vi "Submodule EOL UI.vi"() -> ()   [LabVIEW 2025, in "Submodule EOL.lvlib" / "Submodule EOL.lvclass"]
doc: "Copyright 2017 National Instruments Corporation\n\nLicensed under the Apache License, Version 2.0 (the \"License\"); you may not use this file except in compliance with the License. You may obtain a copy of the License at http://www.apache.org/licenses/LICENSE-2.0\nUnless required by applicable law or agreed to in writing, software distributed under the License is distributed on an \"AS IS\" BASIS, WITHOUT WARRANTIES OR CONDITIONS OF ANY KIND, either express or implied. See the License for the specific language governing permissions and limitations under the License."
uses:
  Submodule EOL.lvclass
  Users/Public/Documents/Sandia National Labs/TSS Plugin/CEF.lvlibp/Node/mainQref.ctl
  Users/Public/Documents/Sandia National Labs/TSS Plugin/CEF.lvlibp/Node/UserEventRef.ctl
  Submodule EOL configuration/Submodule EOL.ctl
  Users/Public/Documents/Sandia National Labs/TSS Plugin/CEF.lvlibp/Node/NodeRef.ctl
  Users/Public/Documents/Sandia National Labs/TSS Plugin/CEF.lvlibp/Node/CEF_Node.lvclass
  C:/Users/Public/Documents/Sandia National Labs/TSS Plugin/CEF.lvlibp/Node/CEF_Node.lvclass
  Users/Public/Documents/Sandia National Labs/TSS Plugin/Abstract Engine.lvlibp/Abstract Instrument/Abstract Instrument.lvclass
  Submodule EOL.lvclass/Submodule EOL.ctl
  Submodule EOL configuration/Submodule EOL configuration.lvclass/Submodule EOL configuration.ctl
  <vilib>/Utility/miscctls.llb/LVPositionTypeDef.ctl
  Users/Public/Documents/Sandia National Labs/TSS Plugin/Engines/DMM.lvlibp/DMM Instrument/DMM Instrument.lvclass
  C:/Users/Public/Documents/Sandia National Labs/TSS Plugin/Abstract Engine.lvlibp/Abstract Instrument/Abstract Instrument.lvclass
  Users/Public/Documents/Sandia National Labs/TSS Plugin/Engines/ACIR.lvlibp/ACIR Instrument/ACIR Instrument.lvclass
  Users/Public/Documents/Sandia National Labs/TSS Plugin/Engines/HiPOT.lvlibp/HiPOT Instrument/HiPOT Instrument.lvclass
  Users/Public/Documents/Sandia National Labs/TSS Plugin/Engines/Digital IO.lvlibp/Digital IO Instrument/Digital IO Instrument.lvclass
  Submodule EOL configuration/Read Submodule EOL.vi
  Submodule EOL configuration/Write Submodule EOL.vi
  Submodule EOL configuration/Submodule EOL configuration.lvclass
panel:
  in  "node ref":T1
  in  "Sequence":cluster{"Sequence":string}
  out "Data":T2 {"HiPOT Channels"."Measurement" format="%#_4p"; "ACIR Channels"."Measurement" format="%#_4p"; "DMM Channels"."Measurement" format="%#_4p"}
  in  "Segmented":enum32{"Setting", "Data", "Sequence"}(radio)
  in  "Submodule EOL":T3={"PLC Folder Names"=[], "Timeout Connect OPC"=0.0, "Connect OPC Trial"=0, "PLC URL"="", "Digitial IO"="", "HiPOT"="", "ACIR with Switch"="", "DMM with Switch"="", "Ignition Folder Names"=[], "Ignition URL"="", "Test Name"="Battery Submodule End of Line"} {"Timeout Connect OPC" format="%#_f"}
  in  "user event":T4
  in  "main queue":T5
  # "ch"
  # "ch"
  # "ch"
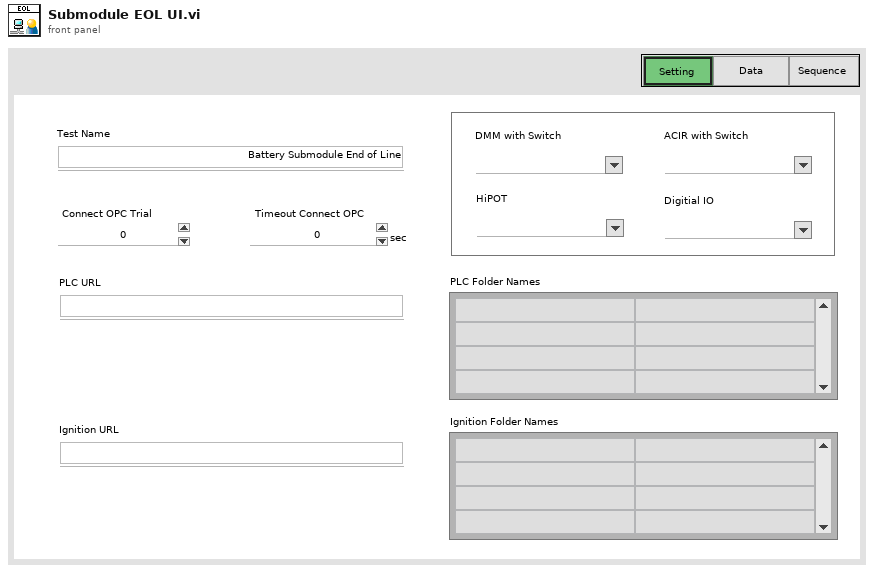
[diagram p1: front panel]
types:
  T1 = typedef "CEF.lvlibp/CEF_Node.lvclass/NodeRef.ctl" = refnum<data-value>
  T2 = cluster{"DMM Channels":cluster{"Channel Alias":string, "Index":i32, "Measurement":dbl}[], "ACIR Channels":cluster{"Channel Alias":string, "Index":i32, "Measurement":dbl}[], "HiPOT Channels":cluster{"Channel Alias":string, "Index":i32, "Measurement":dbl}[], "Digital IO":bool[]}
  T3 = typedef "Submodule EOL.lvlib/Submodule EOL configuration.lvclass/Submodule EOL.ctl" = cluster{"PLC Folder Names":string[][], "Timeout Connect OPC":dbl, "Connect OPC Trial":u32, "PLC URL":string, "Digitial IO":string, "HiPOT":string, "ACIR with Switch":string, "DMM with Switch":string, "Ignition Folder Names":string[][], "Ignition URL":string, "Test Name":string}
  T4 = typedef "CEF.lvlibp/CEF_Node.lvclass/UserEventRef.ctl" = refnum<user-event>
  T5 = typedef "CEF.lvlibp/CEF_Node.lvclass/mainQref.ctl" = refnum<queue>
  T6 = cluster{"Channel Alias":string, "Index":i32, "Measurement":dbl}
  T7 = cluster{"Channel":string, "Index":i32, "Measure":dbl}
  T8 = typedef "LVPositionTypeDef.ctl" = cluster{"Left":i32, "Top":i32}
  T9 = typedef "Abstract Engine.lvlibp/Abstract Instrument.lvclass/Channel.ctl" = cluster{"Alias":string, "DataType":enum16{"Anaolg Input", "Waveform"}, "Unit":enum16{"---", "V", "A", "Ohm", "Hz", "uF", "degC", "deg"}, "Upper limit":dbl, "Lower limit":dbl, "Measurement":variant}
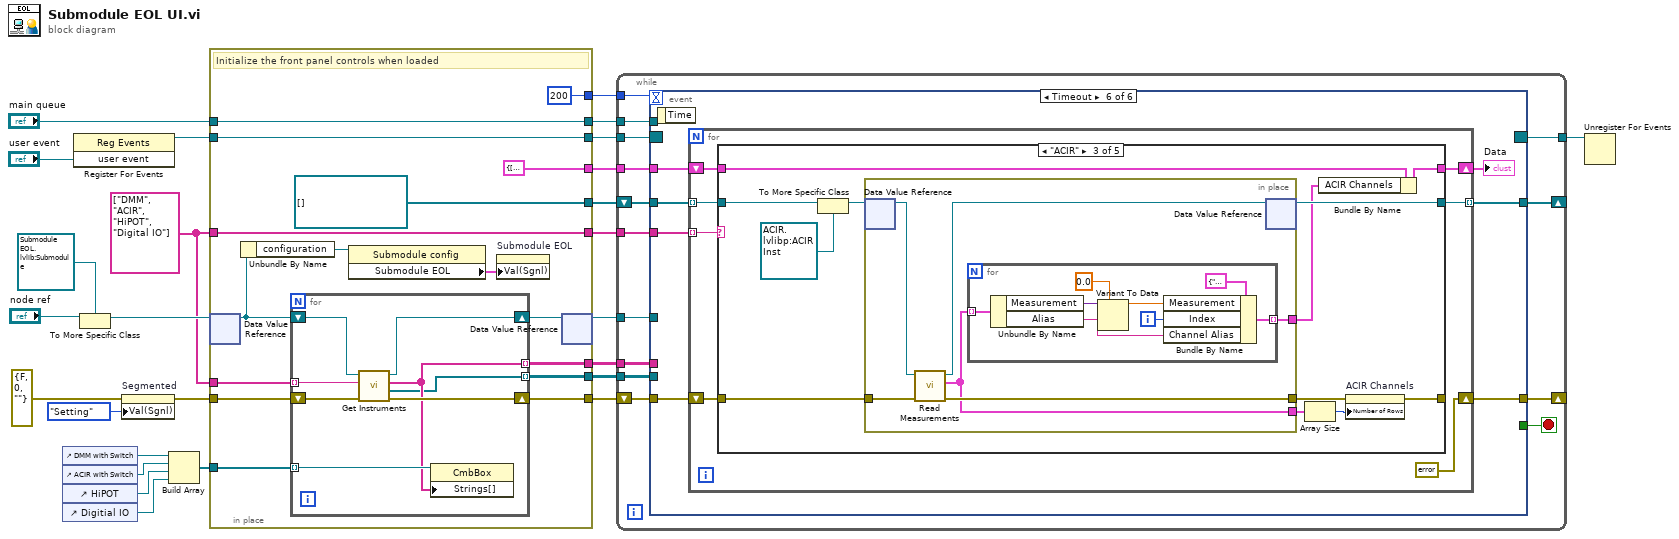
[diagram p0: block diagram]
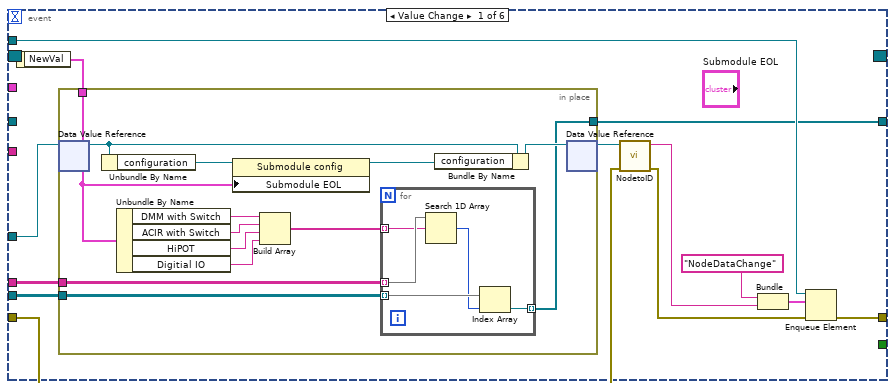
[diagram p2: hidden frame]
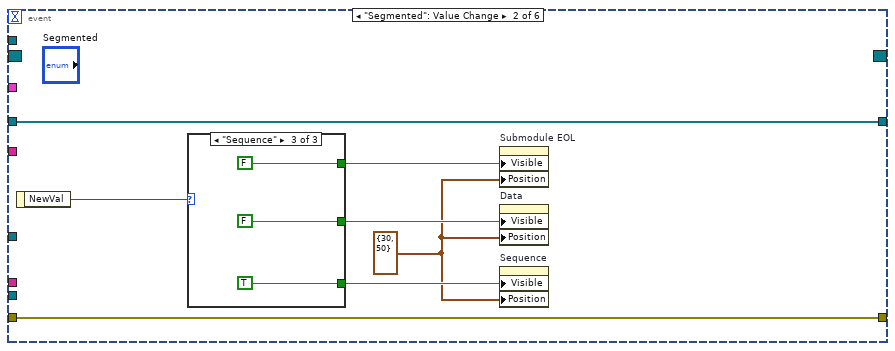
[diagram p3: hidden frame]
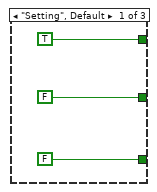
[diagram p4: hidden frame]
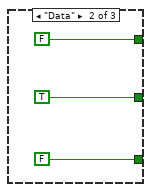
[diagram p5: hidden frame]
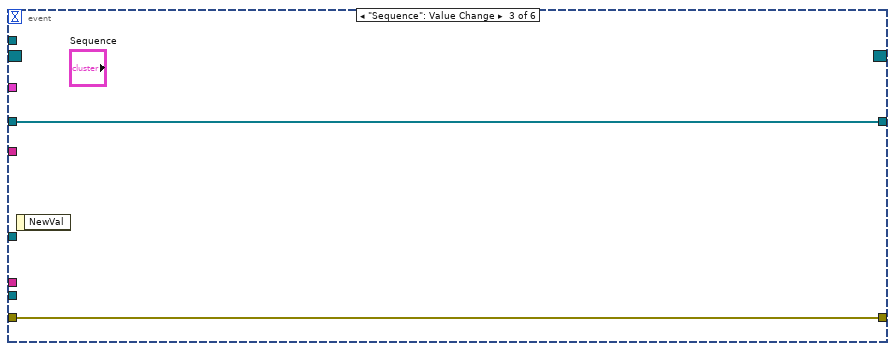
[diagram p6: hidden frame]
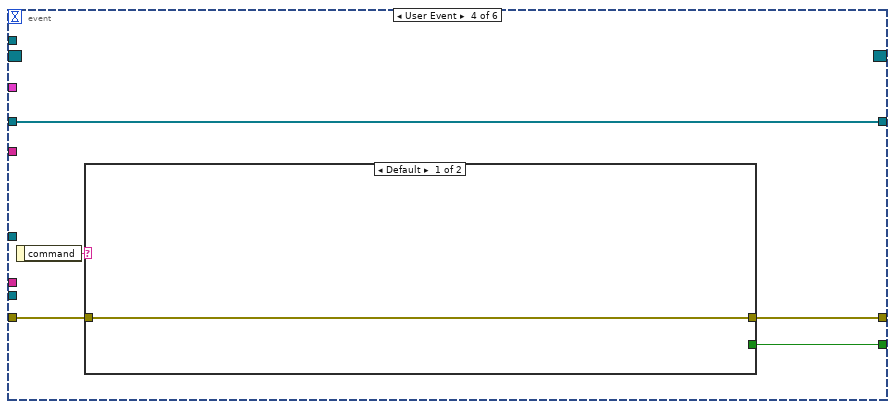
[diagram p7: hidden frame]
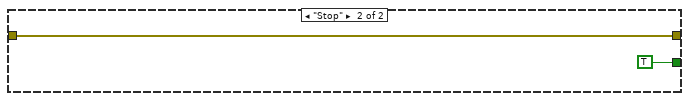
[diagram p8: hidden frame]
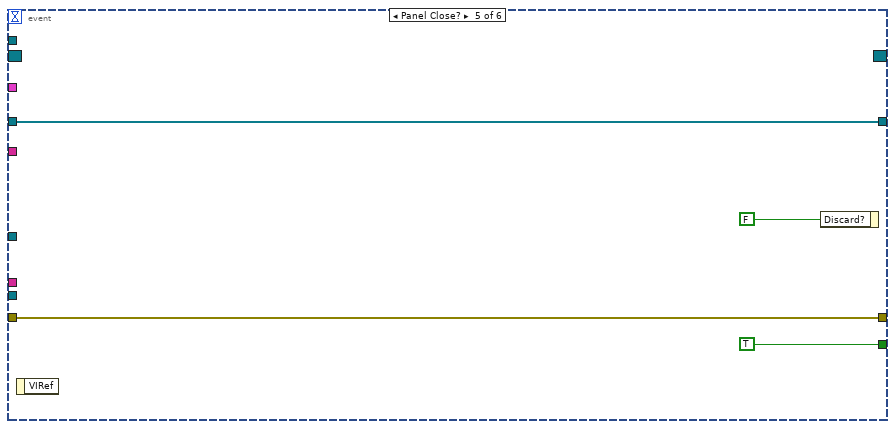
[diagram p9: hidden frame]
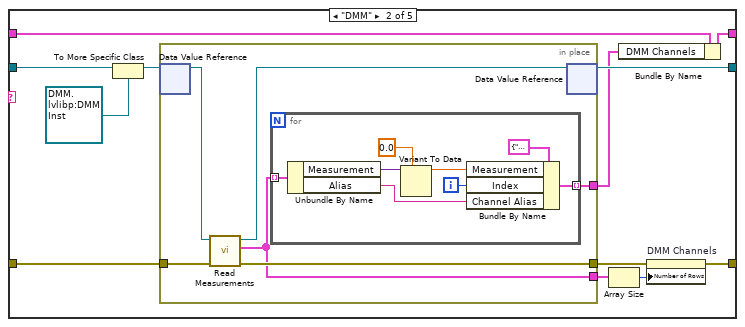
[diagram p11: hidden frame]
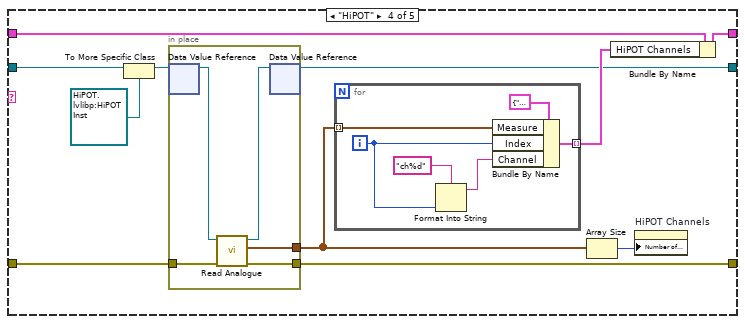
[diagram p12: hidden frame]
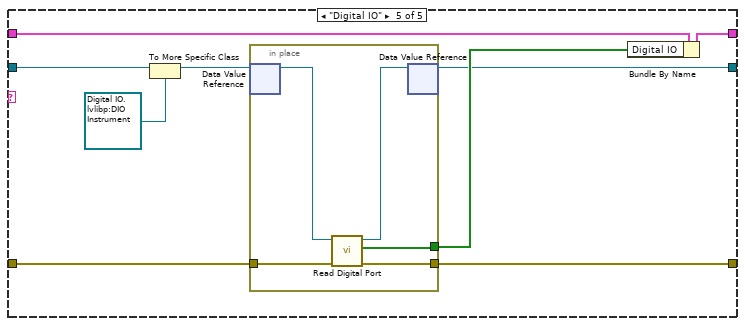
[diagram p13: hidden frame]
diagram:
  w13 = string[] ["DMM", "ACIR", "HiPOT", "Digital IO"]
  n1 = control-ref of="DMM with Switch"() -> (w21:refnum<vi>)
  n2 = control-ref of="ACIR with Switch"() -> (w22:refnum<vi>)
  n3 = control-ref of="HiPOT"() -> (w23:refnum<vi>)
  n4 = control-ref of="Digitial IO"() -> (w24:refnum<vi>)
  n5 = register-events("user event") -> (reference out=w4:refnum<event-registration>)  [unwired: 2 in, 1 out]
  n6 = To More Specific Class(target class=refnum<data-value> refnum ("data value reference"), reference="node ref") -> (specific class reference=w15:refnum<data-value>)  [unwired: 1 in, 1 out]
  n7 = property on="Segmented" class="RadioBtnsControl (strict)"(error in=errorcluster {"status"=FALSE, "code"=0, "source"=""} ("error out"), "Val(Sgnl)"=enum32{"Setting", "Data", "Sequence"}."Setting" ("Segmented Control")) -> (error out=w8:errorcluster)  [unwired: 1 in, 1 out]
  n8 = Build Array(w21, w22, w23, w24) -> (w20:refnum<vi>[])
  n9 = in-place {
    in-place-border: w13 -> [w39]
    in-place-border: w20 -> [w41]
    in-place-border: [w32] -> w6
    in-place-border: "main queue" -> [w40]
    in-place-border: [w40] -> w18
    in-place-border: [w38] -> w17
    in-place-border: [w37] -> w16
    in-place-border: w8 -> [w36]
    in-place-border: [refnum<data-value>[] []] -> w14
    in-place-border: w13 -> [w29]
    in-place-border: [w29] -> w7
    in-place-border: [200] -> w12
    in-place-border: [T2 {"DMM Channels"=[], "ACIR Channels"=[], "HiPOT Channels"=[], "Digital IO"=[]} ("Data")] -> w11
    in-place-border: w4 -> [w30]
    in-place-border: [w30] -> w3
    # "Initialize the front panel controls when loaded"
    n10 = in-place-dvr #1(w15) -> (w28:refnum<class "Submodule EOL.lvclass">)  [unwired: 1 out]
    n11 = Unbundle By Name(w28) -> ("configuration"=w42:refnum<class "Submodule EOL configuration.lvclass">)
    n12 = for {
      shift-right: [w45] -> w32
      shift-left: w36 -> [w46]
      tunnel: w39 -> [w47] mode=indexing
      tunnel: w41 -> [w50] mode=indexing
      tunnel: [w43] -> w38 mode=indexing
      tunnel: [w44] -> w37 mode=indexing
      shift-right: [w48] -> w27
      shift-left: w28 -> [w49]
      n13 = call "Get Instruments.vi"("error in"=w46, "Engine"=w47, "Submodule in"=w49) -> ("error out"=w45:errorcluster, "Instrument nodes"=w43:refnum<data-value>[], "Instruments"=w44:string[], "Submodule out"=w48:refnum<class "Submodule EOL.lvclass">)  [unwired: 5 in]
      n14 = property class="CmbBox"(reference=w50, "Strings[]"=w44) -> ()  [unwired: 1 in, 2 out]
    }
    n15 = property class="Submodule config"(reference=w42) -> ("Submodule EOL"=w31:T3)  [unwired: 1 in, 2 out]
    n16 = property on="Submodule EOL" class="Clust (strict)"("Val(Sgnl)"=w31) -> ()  [unwired: 2 in, 2 out]
    n17 = in-place-dvr #1(w27) -> (w26:refnum<data-value>)  [unwired: 1 out]
  }
  n18 = while {
    tunnel: w3 -> [w58]
    tunnel: w18 -> [w60]
    tunnel: w26 -> [w62]
    tunnel: [w59] -> w25
    shift-right: [w63] -> _
    shift-left: w6 -> [w64]
    tunnel: w17 -> [w57]
    tunnel: w16 -> [w56]
    shift-right: [w55] -> _
    shift-left: w14 -> [w54]
    tunnel: w12 -> [w53]
    tunnel: w11 -> [w52]
    tunnel: w7 -> [w51]
    stop <- w61 stop-if-true
    n19 = event shown="[5] Timeout" {
      selector: w58 -> [_ _ _ _ _ _]
      dyn-events: [_ _ _ _ _ _] -> w59
      timeout: w53 -> [_ _ _ _ _ _]
      tunnel: w64 -> [w65 w100 w113 w116 w125 w131]
      tunnel: [w75 w100 w113 w115 w125 w129] -> w63
      tunnel: w62 -> [w77 _ _ _ _ _]
      tunnel: [_ _ _ w117 TRUE _] -> w61
      tunnel: w60 -> [w72 _ _ _ _ _]
      tunnel: w57 -> [w69 _ _ _ _ _]
      tunnel: w56 -> [w68 _ _ _ _ _]
      tunnel: [w66 w102 w112 w114 w122 w128] -> w55
      tunnel: w54 -> [_ w102 w112 w114 w122 w132]
      tunnel: w52 -> [_ _ _ _ _ w127]
      tunnel: w51 -> [_ _ _ _ _ w126]
      event Value Change {
        n20 = event-data() -> ("NewVal"=w74:T3)  [unwired: 1 out]
        n21 = in-place {
          in-place-border: w74 -> [w86]
          in-place-border: w69 -> [w85]
          in-place-border: w68 -> [w84]
          in-place-border: [w78] -> w66
          # "Initialize the front panel controls when loaded"
          n22 = in-place-dvr #2(w77) -> (w87:refnum<class "Submodule EOL.lvclass">)  [unwired: 1 out]
          n23 = Unbundle By Name(w87) -> ("configuration"=w88:refnum<class "Submodule EOL configuration.lvclass">)
          n24 = Unbundle By Name(w86) -> ("DMM with Switch"=w83:string, "ACIR with Switch"=w82:string, "HiPOT"=w81:string, "Digitial IO"=w80:string)
          n25 = property class="Submodule config"(reference=w88, "Submodule EOL"=w86) -> (reference out=w89:refnum<class "Submodule EOL configuration.lvclass">)  [unwired: 1 in, 1 out]
          n26 = Build Array(w83, w82, w81, w80) -> (w79:string[])
          n27 = for {
            tunnel: w85 -> [w95] mode=indexing
            tunnel: w79 -> [w93] mode=indexing
            tunnel: w84 -> [w94] mode=indexing
            tunnel: [w91] -> w78 mode=indexing
            n28 = Search 1D Array(1D array=w94, element=w93) -> (index of element=w92:i32)  [unwired: 1 in]
            n29 = Index Array(array=w95, index=w92) -> (element=w91:refnum<data-value>)
          }
          n30 = Bundle By Name(cluster=w87, "configuration"=w89) -> (w90:refnum<class "Submodule EOL.lvclass">)
          n31 = in-place-dvr #2(w90) -> (w73:refnum<data-value>)  [unwired: 1 out]
        }
        n32 = call "NodetoID.vi"("error in"=w65, "node ref"=w73) -> ("error out"=w76:errorcluster, "ID"=w71:string)  [unwired: 8 in]
        n33 = Bundle("Message Name"="NodeDataChange", "ID"=w71) -> (w70:cluster{"Message Name":string, "ID":string})  [unwired: 1 in]
        n34 = Enqueue Element(queue=w72, element=w70, error in (no error)=w76) -> (error out=w75:errorcluster)  [unwired: 1 in, 2 out]
      }
      event "Segmented": Value Change {
        w96 = T8 {"Left"=30, "Top"=50} ("Position")
        n35 = event-data() -> ("NewVal"=w101:enum32{"Setting", "Data", "Sequence"})  [unwired: 1 out]
        n36 = case shown="\"Sequence\"" w101 {
          tunnel: [FALSE ("Visible") TRUE ("Visible") FALSE ("Visible")] -> w98
          tunnel: [TRUE ("Visible") FALSE ("Visible") FALSE ("Visible")] -> w99
          tunnel: [FALSE ("Visible") FALSE ("Visible") TRUE ("Visible")] -> w97
          frame "Setting", Default {
          }
          frame "Data" {
          }
          frame "Sequence" {
          }
        }
        n37 = property on="Submodule EOL" class="Clust (strict)"("Visible"=w99, "Position"=w96) -> ()  [unwired: 2 in, 2 out]
        n38 = property on="Data" class="Clust (strict)"("Visible"=w98, "Position"=w96) -> ()  [unwired: 2 in, 2 out]
        n39 = property on="Sequence" class="Clust (strict)"("Visible"=w97, "Position"=w96) -> ()  [unwired: 2 in, 2 out]
      }
      event "Sequence": Value Change {
        n40 = event-data() -> ()  [unwired: 2 out]
      }
      event User Event {
        n41 = event-data() -> ("command"=w118:string)  [unwired: 1 out]
        n42 = case shown="Default" w118 {
          tunnel: [_ TRUE] -> w117
          tunnel: w116 -> [w119 w120]
          tunnel: [w119 w120] -> w115
          frame Default {
          }
          frame "Stop" {
          }
        }
      }
      event Panel Close? {
        n43 = event-data() -> ()  [unwired: 2 out]
        n44 = event-data("Discard?"=FALSE) -> ()  [unwired: 1 in, 1 out]
      }
      event Timeout {
        n45 = event-data() -> ()  [unwired: 2 out]
        n46 = for {
          tunnel: w132 -> [w138] mode=indexing
          tunnel: w126 -> [w139] mode=indexing
          shift-right: [errorcluster {"status"=FALSE, "code"=0, "source"=""} ("error out")] -> w129
          shift-left: w131 -> [w137]
          shift-right: [w136] -> w130
          shift-left: w127 -> [w135]
          tunnel: [w134] -> w128 mode=indexing
          n47 = case shown="\"ACIR\"" w139 {
            tunnel: w138 -> [w140 w153 w179 w204 w224]
            tunnel: w137 -> [w142 w147 w174 w196 w218]
            tunnel: [w142 w145 w171 w202 w222] -> _
            tunnel: [w141 w150 w176 w198 w220] -> w136
            tunnel: w135 -> [w141 w149 w175 w197 w219]
            tunnel: [w140 w148 w173 w195 w217] -> w134
            frame Default {
            }
            frame "DMM" {
              n48 = To More Specific Class(target class=refnum<data-value> refnum, reference=w153) -> (specific class reference=w154:refnum<data-value>)  [unwired: 1 in, 1 out]
              n49 = in-place {
                in-place-border: w147 -> [w159]
                in-place-border: [w157] -> w146
                in-place-border: [w155] -> w144
                in-place-border: [w156] -> w143
                n50 = in-place-dvr #3(w154) -> (w160:refnum<class "DMM Instrument.lvclass">)  [unwired: 1 out]
                n51 = call-dynamic "Read Measurements.vi"("error in"=w159, "DMM Instrument"=w160) -> ("error out"=w157:errorcluster, "Measurements"=w155:T9[], "DMM Instrument out"=w158:refnum<class "DMM Instrument.lvclass">)  [unwired: 7 in]
                n52 = for {
                  tunnel: [w168] -> w156 mode=indexing
                  tunnel: w155 -> [w166] mode=indexing
                  i -> [w162]
                  n53 = Unbundle By Name(w166) -> ("Measurement"=w164:variant, "Alias"=w161:string)
                  n54 = Variant To Data(type=0.0 ("Measurement"), Variant=w164) -> (data=w163:dbl)  [unwired: 1 in, 1 out]
                  n55 = Bundle By Name(cluster=T6 {"Channel Alias"="", "Index"=0, "Measurement"=0.0} ("Channel"), "Measurement"=w163, "Index"=w162, "Channel Alias"=w161) -> (w168:T6)
                }
                n56 = in-place-dvr #3(w158) -> (w148:refnum<data-value>)  [unwired: 1 out]
              }
              n57 = Array Size(array=w144) -> (size(s)=w151:i32)
              n58 = Bundle By Name(cluster=w149, "DMM Channels"=w143) -> (w150:T2)
              n59 = property on="DMM Channels" class="Arr (strict)"(error in=w146, "Number of Rows"=w151) -> (error out=w145:errorcluster)  [unwired: 1 in, 1 out]
            }
            frame "ACIR" {
              n60 = To More Specific Class(target class=refnum<data-value> refnum, reference=w179) -> (specific class reference=w180:refnum<data-value>)  [unwired: 1 in, 1 out]
              n61 = in-place {
                in-place-border: [w184] -> w172
                in-place-border: w174 -> [w186]
                in-place-border: [w181] -> w169
                in-place-border: [w182] -> w170
                n62 = in-place-dvr #4(w180) -> (w185:refnum<class "ACIR Instrument.lvclass">)  [unwired: 1 out]
                n63 = call-dynamic "Read Measurements.vi"("error in (no error)"=w186, "ACIR Instrument in"=w185) -> ("error out"=w184:errorcluster, "Measurements"=w181:T9[], "ACIR Instrument out"=w183:refnum<class "ACIR Instrument.lvclass">)  [unwired: 7 in]
                n64 = for {
                  tunnel: [w194] -> w182 mode=indexing
                  tunnel: w181 -> [w192] mode=indexing
                  i -> [w188]
                  n65 = Unbundle By Name(w192) -> ("Measurement"=w190:variant, "Alias"=w187:string)
                  n66 = Variant To Data(type=0.0 ("Measurement"), Variant=w190) -> (data=w189:dbl)  [unwired: 1 in, 1 out]
                  n67 = Bundle By Name(cluster=T6 {"Channel Alias"="", "Index"=0, "Measurement"=0.0} ("Channel"), "Measurement"=w189, "Index"=w188, "Channel Alias"=w187) -> (w194:T6)
                }
                n68 = in-place-dvr #4(w183) -> (w173:refnum<data-value>)  [unwired: 1 out]
              }
              n69 = Array Size(array=w169) -> (size(s)=w177:i32)
              n70 = Bundle By Name(cluster=w175, "ACIR Channels"=w170) -> (w176:T2)
              n71 = property on="ACIR Channels" class="Arr (strict)"(error in=w172, "Number of Rows"=w177) -> (error out=w171:errorcluster)  [unwired: 1 in, 1 out]
            }
            frame "HiPOT" {
              n72 = To More Specific Class(target class=refnum<data-value> refnum, reference=w204) -> (specific class reference=w205:refnum<data-value>)  [unwired: 1 in, 1 out]
              n73 = in-place {
                in-place-border: w196 -> [w215]
                in-place-border: [w214] -> w202
                in-place-border: [w213] -> w201
                n74 = in-place-dvr #5(w205) -> (w216:refnum<class "HiPOT Instrument.lvclass">)  [unwired: 1 out]
                n75 = call-dynamic "Read Analogue.vi"("error in (no error)"=w215, "HiPOT Instrument"=w216) -> ("error out"=w214:errorcluster, "Waveforms"=w213:waveform(dbl)[], "HiPOT Instrument out"=w212:refnum<class "HiPOT Instrument.lvclass">)  [unwired: 7 in]
                n76 = in-place-dvr #5(w212) -> (w195:refnum<data-value>)  [unwired: 1 out]
              }
              n77 = for {
                tunnel: [w211] -> w199 mode=indexing
                tunnel: w201 -> [w210] mode=indexing
                i -> [w207]
                n78 = Format Into String(format string="ch%d", w207) -> (resulting string=w206:string)  [unwired: 2 in, 1 out]
                n79 = Bundle By Name(cluster=T7 {"Channel"="", "Index"=0, "Measure"=0.0} ("Channel"), "Measure"=w210, "Index"=w207, "Channel"=w206) -> (w211:T7)
              }
              n80 = Array Size(array=w201) -> (size(s)=w200:i32)
              n81 = Bundle By Name(cluster=w197, "HiPOT Channels"=w199) -> (w198:T2)
              n82 = property on="HiPOT Channels" class="Arr (strict)"("Number of Columns"=w200) -> ()  [unwired: 2 in, 2 out]
            }
            frame "Digital IO" {
              n83 = To More Specific Class(target class=refnum<data-value> refnum, reference=w224) -> (specific class reference=w225:refnum<data-value>)  [unwired: 1 in, 1 out]
              n84 = in-place {
                in-place-border: w218 -> [w228]
                in-place-border: [w227] -> w222
                in-place-border: [w226] -> w221
                n85 = in-place-dvr #6(w225) -> (w230:refnum<class "Digital IO Instrument.lvclass">)  [unwired: 1 out]
                n86 = call-dynamic "Read Digital Port.vi"("error in (no error)"=w228, "Digital IO Instrumentgital Input in"=w230) -> ("error out"=w227:errorcluster, "DIs"=w226:bool[], "Digital IO Instrumentgital Input out"=w229:refnum<class "Digital IO Instrument.lvclass">)  [unwired: 7 in]
                n87 = in-place-dvr #6(w229) -> (w217:refnum<data-value>)  [unwired: 1 out]
              }
              n88 = Bundle By Name(cluster=w219, "Digital IO"=w221) -> (w220:T2)
            }
          }
        }
        "Data" <- w130
      }
    }
  }
  n89 = Unregister For Events(event registration refnum=w25) -> ()  [unwired: 1 in, 1 out]
